vi "HFRR ADV v09 new software.vi"() -> ()   [LabVIEW 2025] (continued)
                        n2272 = local read "EVENT LOG"() -> (w3332:string)
                        n2273 = call "Event Log.vi"("Content"=w3330, "EVENT LOG"=w3332) -> ("EVENT LOG"=w3331:string)  [unwired: 8 in, 1 out]
                        n2274 = local write "EVENT LOG"(w3331) -> ()
                      }
                      frame #22 {
                        n2275 = Wait (ms)(milliseconds to wait=u32 50) -> ()  [unwired: 1 out]
                      }
                      frame #23 {
                        n2276 = local read "NORMAL LOAD"() -> (w3335:dbl)
                        n2277 = Number To Fractional String(number=w3335, precision (6)=i16 2) -> (F-format string=w3336:string)  [unwired: 2 in]
                        n2278 = Concatenate Strings("Applied Load [grams] :" ("Content"), w3336) -> (w3338:string)
                        n2279 = local read "EVENT LOG"() -> (w3340:string)
                        n2280 = call "Event Log.vi"("Content"=w3338, "EVENT LOG"=w3340) -> ("EVENT LOG"=w3339:string)  [unwired: 8 in, 1 out]
                        n2281 = local write "EVENT LOG"(w3339) -> ()
                      }
                      frame #24 {
                        n2282 = Wait (ms)(milliseconds to wait=u32 50) -> ()  [unwired: 1 out]
                      }
                      frame #25 {
                        n2283 = local read "Set Strk"() -> (w3343:dbl)
                        n2284 = Number To Fractional String(number=w3343, precision (6)=i16 2) -> (F-format string=w3344:string)  [unwired: 2 in]
                        n2285 = Concatenate Strings("Set Stroke [mm] :" ("Content"), w3344) -> (w3346:string)
                        n2286 = local read "EVENT LOG"() -> (w3348:string)
                        n2287 = call "Event Log.vi"("Content"=w3346, "EVENT LOG"=w3348) -> ("EVENT LOG"=w3347:string)  [unwired: 8 in, 1 out]
                        n2288 = local write "EVENT LOG"(w3347) -> ()
                      }
                      frame #26 {
                        n2289 = Wait (ms)(milliseconds to wait=u32 50) -> ()  [unwired: 1 out]
                      }
                      frame #27 {
                        n2290 = local read "Set Temp"() -> (w3351:dbl)
                        n2291 = Number To Fractional String(number=w3351, precision (6)=i16 2) -> (F-format string=w3352:string)  [unwired: 2 in]
                        n2292 = Concatenate Strings("Set Temperature [deg C] :" ("Content"), w3352) -> (w3354:string)
                        n2293 = local read "EVENT LOG"() -> (w3356:string)
                        n2294 = call "Event Log.vi"("Content"=w3354, "EVENT LOG"=w3356) -> ("EVENT LOG"=w3355:string)  [unwired: 8 in, 1 out]
                        n2295 = local write "EVENT LOG"(w3355) -> ()
                      }
                      frame #28 {
                        n2296 = Wait (ms)(milliseconds to wait=u32 50) -> ()  [unwired: 1 out]
                      }
                      frame #29 {
                        n2297 = local read "Set Rh"() -> (w3359:dbl)
                        n2298 = Number To Fractional String(number=w3359, precision (6)=i16 2) -> (F-format string=w3360:string)  [unwired: 2 in]
                        n2299 = Concatenate Strings("Set Humidity [%RH] :" ("Content"), w3360) -> (w3362:string)
                        n2300 = local read "EVENT LOG"() -> (w3364:string)
                        n2301 = call "Event Log.vi"("Content"=w3362, "EVENT LOG"=w3364) -> ("EVENT LOG"=w3363:string)  [unwired: 8 in, 1 out]
                        n2302 = local write "EVENT LOG"(w3363) -> ()
                      }
                      frame #30 {
                        n2303 = Wait (ms)(milliseconds to wait=u32 50) -> ()  [unwired: 1 out]
                      }
                      frame #31 {
                        n2304 = local read "test time"() -> (w3367:dbl)
                        n2305 = Number To Fractional String(number=w3367, precision (6)=i16 1) -> (F-format string=w3368:string)  [unwired: 2 in]
                        n2306 = Concatenate Strings("Test Duration [mins] :" ("Content"), w3368) -> (w3370:string)
                        n2307 = local read "EVENT LOG"() -> (w3372:string)
                        n2308 = call "Event Log.vi"("Content"=w3370, "EVENT LOG"=w3372) -> ("EVENT LOG"=w3371:string)  [unwired: 8 in, 1 out]
                        n2309 = local write "EVENT LOG"(w3371) -> ()
                      }
                      frame #32 {
                        w3373 = dbl[] [] ("History Data")
                        w3374 = cluster{"y":dbl, dbl, "y":dbl}[] [] ("History Data")
                        w3375 = FALSE ("Visible")
                        n2310 = property on="Stroke ( mm )" class="WFChart (strict)"("History Data"=w3374) -> ()  [unwired: 2 in, 2 out]
                        n2311 = property on="Humidity ( %RH )" class="WFChart (strict)"("History Data"=w3373) -> ()  [unwired: 2 in, 2 out]
                        n2312 = property on="Temperature ( Deg C )" class="WFChart (strict)"("History Data"=w3373) -> ()  [unwired: 2 in, 2 out]
                        n2313 = property on="Electrical Contact Resistance ( % )" class="WFChart (strict)"("History Data"=w3373) -> ()  [unwired: 2 in, 2 out]
                        n2314 = property on="Coefficient of Friction" class="WFChart (strict)"("History Data"=w3373) -> ()  [unwired: 2 in, 2 out]
                        n2315 = property on="Frictional Force ( N )" class="WFChart (strict)"("History Data"=w3373) -> ()  [unwired: 2 in, 2 out]
                        n2316 = property on="Coefficient of Friction" class="WFChart (strict)"("History Data"=w3373) -> ()  [unwired: 2 in, 2 out]
                        n2317 = property on="Frictional Force ( N )" class="WFChart (strict)"("History Data"=w3373) -> ()  [unwired: 2 in, 2 out]
                        n2318 = property on="Electrical Contact Resistance ( % )" class="WFChart (strict)"("History Data"=w3373) -> ()  [unwired: 2 in, 2 out]
                        n2319 = property on="Humidity ( %RH )" class="WFChart (strict)"("History Data"=w3373) -> ()  [unwired: 2 in, 2 out]
                        n2320 = property on="Stroke ( mm )" class="WFChart (strict)"("History Data"=w3374) -> ()  [unwired: 2 in, 2 out]
                        n2321 = property on="Temperature ( Deg C )" class="WFChart (strict)"("History Data"=w3373) -> ()  [unwired: 2 in, 2 out]
                        n2322 = property on="Service Password Log" class="Str"("Visible"=w3375) -> ()  [unwired: 2 in, 2 out]
                        n2323 = property on="Password 3" class="Clust (strict)"("Visible"=w3375) -> ()  [unwired: 2 in, 2 out]
                      }
                    }
                    "TEST FILE NAM,E SAVED" <- TRUE ("TEST FILE NAM,E SAVED")
                  }
                }
              }
            }
          }
        }
        n2324 = case shown="True" w2679 {
          frame False {
            n2325 = local write "tfalg"(0.0 ("tfalg")) -> ()
          }
          frame True {
            n2326 = local read "tfalg"() -> (w2824:dbl)
            n2327 = Equal?(x=w2824, y=0.0) -> (x = y?=w2825:bool)
            n2328 = case shown="True" w2825 {
              frame False {
              }
              frame True {
                n2329 = local read "Total No. of Tests"() -> (w2828:dbl)
                n2330 = local write "tfalg"(1.0 ("tfalg")) -> ()
                n2331 = local write "acq 2"(FALSE ("acq 2")) -> ()
                n2332 = Wait (ms)(milliseconds to wait=u32 200) -> ()  [unwired: 1 out]
                n2333 = Increment(x=w2828) -> (x+1=w2827:dbl)
                n2334 = local write "Total No. of Tests"(w2827) -> ()
              }
            }
          }
        }
        n2335 = local write "Test \nStatus"(w2685) -> ()
        n2336 = local write "Save"(w2685) -> ()
        n2337 = local read "Main Tab"() -> (w2642:T2)
        n2338 = case shown="True" w2666 {
          tunnel: [FALSE ("RUN") TRUE ("RUN")] -> w2665
          tunnel: [_ 1] -> w2658
          frame False {
          }
          frame True {
          }
        }
        n2339 = In Range and Coerce(upper limit=w2673, x=w2646, lower limit=w2672) -> (In Range?=w2664:bool)  [unwired: 1 out]
        n2340 = In Range and Coerce(upper limit=w2670, x=w2645, lower limit=w2671) -> (In Range?=w2662:bool)  [unwired: 1 out]
        n2341 = case shown="True" w2678 {
          frame False {
            n2342 = local read "Rt 3"() -> (w2806:bool)
            n2343 = case shown="True" w2806 {
              frame False {
              }
              frame True {
                n2344 = local write "Rt 3"(FALSE ("Rt 3")) -> ()
                n2345 = local write "Json End Flg"(TRUE ("Upld AR 2")) -> ()
              }
            }
            "Rt" <- TRUE ("Rt")
            "Rt 2" <- FALSE ("Rt")
          }
          frame True {
            n2346 = local read "Rt"() -> (w2813:bool)
            n2347 = local write "Rt 2"(TRUE ("Rt 2")) -> ()
            n2348 = case shown="True" w2813 {
              frame False {
              }
              frame True {
                w2814 = TRUE ("Upld AR 2")
                n2349 = local write "Rt"(FALSE ("Rt")) -> ()
                n2350 = local write "Upld AR"(w2814) -> ()
                n2351 = local write "Json St Flg"(w2814) -> ()
              }
            }
            "Rt 3" <- TRUE ("Rt 3")
          }
        }
        n2352 = case shown="True" w2664 {
          tunnel: [FALSE ("RUN") TRUE ("RUN")] -> w2663
          tunnel: [_ 2] -> w2657
          frame False {
          }
          frame True {
          }
        }
        n2353 = case shown="True" w2662 {
          tunnel: [FALSE ("RUN") TRUE ("RUN")] -> w2661
          tunnel: [_ 3] -> w2656
          frame False {
          }
          frame True {
          }
        }
        n2354 = case shown="\"Acquire\"" w2642 {
          tunnel: w2644 -> [_ w2875]
          frame Default {
            w2874 = 0.0 ("output")
            n2355 = local write "PID-out"(w2874) -> ()
            n2356 = local write "Frequency ( Hz )"(w2874) -> ()
          }
          frame "Acquire" {
            n2357 = stacked-sequence {
              frame #0 {
                n2358 = local read "Auto Start Test"() -> (w2877:bool)
                n2359 = case shown="True" w2877 {
                  tunnel: "RUN" -> [w2898 w2901]
                  tunnel: [w2898 w2900] -> w2878
                  frame False {
                  }
                  frame True {
                    n2360 = local read "Auto Start Temp"() -> (w2899:bool)
                    n2361 = Or(x=w2901, y=w2899) -> (x .or. y?=w2900:bool)
                  }
                }
                n2362 = local read "clk"() -> (w2897:dbl)
                n2363 = local read "Save"() -> (w2893:bool)
                n2364 = Equal?(x=w2897, y=0.0) -> (x = y?=w2894:bool)
                n2365 = And(x=w2894, y=w2893) -> (x .and. y?=w2895:bool)
                n2366 = Not(x="Engage") -> (.not. x?=w2884:bool)
                n2367 = case shown="True" w2878 {
                  tunnel: [0.0 w2919] -> w2880
                  frame False {
                    (unwired) TRUE ("Visible")
                    n2368 = local read "Auto Start Test"() -> (w2905:bool)
                    n2369 = local write "Start Time"(TRUE ("Start Time")) -> ()
                    n2370 = property on="Stroke 2" class="DigNum (strict)"("Visible"=FALSE) -> ()  [unwired: 2 in, 2 out]
                    n2371 = case shown="False" w2905 {
                      frame False {
                        n2372 = property on="Heater Button" class="Bool (strict)"("DisabledEnum"=T17."Enabled" ("Disabled")) -> ()  [unwired: 2 in, 2 out]
                        n2373 = property on="Humidity" class="Bool (strict)"("DisabledEnum"=T17."Enabled" ("Disabled")) -> ()  [unwired: 2 in, 2 out]
                      }
                      frame True {
                      }
                    }
                    n2374 = case shown="False" "TestCompFlg" {
                      frame False {
                        n2375 = local read "StartFlg"() -> (w2913:bool)
                        n2376 = case shown="True" w2913 {
                          frame False {
                          }
                          frame True {
                            n2377 = flat-sequence {
                              frame #0 {
                                n2378 = local read "EVENT LOG"() -> (w2915:string)
                                n2379 = call "Event Log.vi"("Content"="Test was interrupted", "EVENT LOG"=w2915) -> ("EVENT LOG"=w2916:string)  [unwired: 8 in, 1 out]
                                n2380 = local write "EVENT LOG"(w2916) -> ()
                              }
                              frame #1 {
                                w2918 = FALSE ("StartFlg")
                                n2381 = property on="Heater Button" class="Bool (strict)"("Val(Sgnl)"=FALSE ("Value (Signaling)")) -> ()  [unwired: 2 in, 2 out]
                                n2382 = local write "Heater Button"(w2918) -> ()
                                n2383 = local write "StartFlg"(w2918) -> ()
                                n2384 = local write "Humidity"(w2918) -> ()
                              }
                            }
                          }
                        }
                      }
                      frame True {
                      }
                    }
                    n2385 = local write "String 14"("Test will autostart once parameters reach the set value." ("String 14")) -> ()
                  }
                  frame True {
                    (unwired) FALSE ("Visible")
                    n2386 = property on="Stroke 2" class="DigNum (strict)"("Visible"=TRUE) -> ()  [unwired: 2 in, 2 out]
                    n2387 = property on="STOP 2" class="Bool (strict)"("Disabled"=u8 2) -> ()  [unwired: 2 in, 2 out]
                    n2388 = local write "String 14"(" Running....." ("String 14")) -> ()
                    n2389 = property on="Heater Button" class="Bool (strict)"("DisabledEnum"=T17."Disabled and Grayed Out" ("Disabled")) -> ()  [unwired: 2 in, 2 out]
                    n2390 = property on="Humidity" class="Bool (strict)"("DisabledEnum"=T17."Disabled and Grayed Out" ("Disabled")) -> ()  [unwired: 2 in, 2 out]
                    n2391 = case shown="True" "Start Time" {
                      selector: "Start Time" -> [_ w2938]
                      frame False {
                      }
                      frame True {
                        n2392 = Not(x=w2938) -> (.not. x?=w2937:bool)
                        n2393 = local write "Start Time"(w2937) -> ()
                        n2394 = local read "EVENT LOG"() -> (w2939:string)
                        n2395 = call "Event Log.vi"("Content"="Test in progress", "EVENT LOG"=w2939) -> ("EVENT LOG"=w2941:string)  [unwired: 8 in, 1 out]
                        n2396 = local write "EVENT LOG"(w2941) -> ()
                      }
                    }
                    n2397 = disable-structure shown="Enabled" {
                      disable-tunnel: [w2930 w2936] -> w2919
                      frame Disabled {
                        n2398 = local read "Set Hz"() -> (w2933:dbl)
                        n2399 = call <vilib>:"Uniform White Noise Waveform.vi"() -> ("signal out"=w2932:waveform(dbl))  [unwired: 10 in, 1 out]
                        n2400 = Random Number (0-1)() -> (number: 0 to 1=w2929:dbl)
                        n2401 = Add(x=w2933, y=w2932) -> (x+y=w2931:waveform(dbl))
                        n2402 = Multiply(x=ext 0.01 ("y"), y=w2929) -> (x*y=w2927:ext)
                        n2403 = Multiply(x=w2931, y=w2927) -> (x*y=w2930:waveform(ext))
                      }
                      frame Enabled {
                        n2404 = call-poly <vilib>:"Random Number (Range).vi"("lower bound (0)"=49.89, "upper bound (100)"=50.8) -> ("number"=w2936:dbl)  [unwired: 9 in]
                      }
                    }
                    "StartFlg" <- TRUE ("StartFlg")
                  }
                }
                n2405 = case shown="True" w2895 {
                  frame False {
                  }
                  frame True {
                    n2406 = local write "clk"(10.0 ("clk")) -> ()
                    n2407 = Get Date/Time In Seconds() -> (seconds since 1Jan1904=w2944:timestamp)
                    n2408 = To Double Precision Float(number=w2944) -> (double precision float=w2942:dbl)
                    n2409 = local write "acq timer"(w2942) -> ()
                    n2410 = local write "act save time"(w2942) -> ()
                  }
                }
                n2411 = call "Elapsed Time"("Time Target (s)"="Countdown", "Reset"=w2884) -> ("Elapsed Time (s)"=w2889:dbl, "Time has Elapsed"=w2887:bool)  [unwired: 10 in, 6 out]
                "Countdown 2" <- w2889
                n2412 = Subtract(x=w2889, y=2.0) -> (x-y=w2892:dbl)
                n2413 = Less?(x=w2892, y="Countdown") -> (x < y?=w2890:bool)
                n2414 = And(x=w2890, y=w2887) -> (x .and. y?=w2886:bool)
                n2415 = case shown="True" w2886 {
                  frame False {
                  }
                  frame True {
                    (unwired) dbl[] [] ("History Data")
                    n2416 = local write "Engage"(FALSE ("Engage")) -> ()
                    n2417 = local write "RUN"(TRUE ("RUN")) -> ()
                    n2418 = local read "Humidity ( %RH )"() -> (→"Rh Before":dbl)
                  }
                }
                n2419 = local read "Test \nStatus"() -> (w2882:bool)
                n2420 = Select(t=w2880, s=w2882, f=0.0) -> (s? t:f=w2881:dbl)
                n2421 = local write "Frequency ( Hz )"(w2881) -> ()
              }
              frame #1 {
                w2967 = 1000000.0 ("x")
                # "HC;1/0\nST;VALUE"
                # "Elapsed time\ncof\nstroke\nAir temp\nTemp\nHumidity"
                # "acq timer\n\nact save time"
                # "convert to microseconds"
                n2422 = local read "COUNT"() -> (w2950:i32)
                n2423 = local read "Rate"() -> (w2963:dbl)
                n2424 = Divide(x=w2967, y=w2963) -> (x/y=w2968:dbl)
                n2425 = Greater Or Equal?(x=w2950, y=250) -> (x >= y?=w2949:bool)
                n2426 = Get Date/Time In Seconds() -> (seconds since 1Jan1904=w2970:timestamp)
                n2427 = case shown="True" w2949 {
                  frame False {
                    n2428 = local read "COUNT"() -> (w2971:i32)
                    n2429 = Increment(x=w2971) -> (x+1=w2972:i32)
                    n2430 = local write "COUNT"(w2972) -> ()
                  }
                  frame True {
                    n2431 = local write "COUNT"(0 ("COUNT")) -> ()
                  }
                }
                n2432 = local read "Samplingtime 2"() -> (w2948:dbl)
                n2433 = local read "act save time"() -> (w2965:dbl)
                n2434 = Divide(x=w2968, y=w2967) -> (x/y=w2966:dbl)
                n2435 = To Double Precision Float(number=w2970) -> (double precision float=w2959:dbl)
                n2436 = Add(x=w2965, y=w2948) -> (x+y=w2964:dbl)
                n2437 = local read "acq timer"() -> (w2969:dbl)
                n2438 = local read "COUNT"() -> (w2952:i32)
                n2439 = Greater Or Equal?(x=w2959, y=w2964) -> (x >= y?=w2947:bool)
                n2440 = Multiply(x=w2966, y=w2952) -> (x*y=w2958:dbl)
                n2441 = Subtract(x=w2959, y=w2969) -> (x-y=w2961:dbl)
                n2442 = local read "Save"() -> (w2962:bool)
                n2443 = Add(x=w2961, y=w2958) -> (x+y=w2945:dbl)
                "Elapsed time 3" <- w2945
                n2444 = And(x=w2947, y=w2962) -> (x .and. y?=w2960:bool)
                n2445 = Divide(x=w2945, y=60.0) -> (x/y=w2956:dbl)
                n2446 = local read "Test \nStatus"() -> (w2946:bool)
                n2447 = local read "clk"() -> (w2953:dbl)
                n2448 = Equal?(x=w2953, y=10.0) -> (x = y?=w2955:bool)
                n2449 = case shown="True" w2960 {
                  tunnel: w2959 -> [_ w3081]
                  tunnel: [FALSE ("Boolean 2") TRUE ("Boolean 2")] -> _
                  frame False {
                  }
                  frame True {
                    w3035 = ";" ("Substring")
                    # "Pid out/\nFreq response value"
                    n2450 = local write "act save time"(w3081) -> ()
                    n2451 = local read "FILE"() -> (w3029:string)
                    n2452 = call "file check.vi"("file name in"=w3029) -> ("error out"=w3032:errorcluster, "file name out"=w3027:string)  [unwired: 9 in]
                    n2453 = call "FILE PATH CREATION.vi"("error in"=w3032, "FILE NAME :"=w3027) -> ("FILE OUT"=w3030:path)  [unwired: 8 in, 1 out]
                    n2454 = Concatenate Strings(w3027, ".dgf" ("Substring")) -> (w3031:string)
                    n2455 = local read "FF 2"() -> (→"Frictional Force ( N )" →"Frictional Force ( N )":dbl)
                    n2456 = Build Path(base path=w3030, name or relative path=w3031) -> (appended path=w3026:path)
                    n2457 = local read "COF 2"() -> (w3040:dbl)
                    "cof" <- w3040
                    "Coefficient of Friction" <- w3040
                    "COF 4" <- w3040
                    "Coefficient of Friction" <- w3040
                    n2458 = local read "LVDT STROKE"() -> (w3024:dbl)
                    n2459 = local read "Add up Stroke"() -> (w3022:dbl)
                    n2460 = local read "TEMP"() -> (w3043:dbl)
                    "Temp" <- w3043
                    "Temperature ( Deg C )" <- w3043
                    n2461 = local read "Humidity ( %RH )"() -> (w3042:dbl)
                    "Humidity ( %RH )" <- w3042
                    "Humidity ( %RH )" <- w3042
                    n2462 = local read "Frequency ( Hz )"() -> (w3049:dbl)
                    n2463 = local read "Elapsed time"() -> (w3074:dbl)
                    n2464 = local read "AIR TEMP"() -> (w3047:dbl)
                    n2465 = local read "PID-out"() -> (w3052:dbl)
                    n2466 = Subtract(x=w3024, y=w3022) -> (x-y=w3023:dbl)
                    n2467 = Absolute Value(x=w3023) -> (abs(x)=w3021:dbl)
                    n2468 = local write "Temperature ( Deg C )"(w3043) -> ()
                    n2469 = Number To Fractional String(number=w3021, width (-)=i16 9 ("precision (6)"), precision (6)=i16 6) -> (F-format string=w3067:string)  [unwired: 1 in]
                    n2470 = Number To Fractional String(number=w3047, width (-)=i16 9 ("precision (6)"), precision (6)=i16 3) -> (F-format string=w3066:string)  [unwired: 1 in]
                    n2471 = Number To Fractional String(number=w3043, width (-)=i16 9 ("precision (6)"), precision (6)=i16 3) -> (F-format string=w3063:string)  [unwired: 1 in]
                    n2472 = Number To Fractional String(number=w3042, width (-)=i16 9 ("precision (6)"), precision (6)=i16 3) -> (F-format string=w3060:string)  [unwired: 1 in]
                    n2473 = Number To Fractional String(number=0.0, width (-)=i16 9 ("precision (6)"), precision (6)=i16 3) -> (F-format string=w3057:string)  [unwired: 1 in]
                    n2474 = Number To Fractional String(number=w3052, width (-)=i16 9 ("precision (6)"), precision (6)=i16 3) -> (F-format string=w3053:string)  [unwired: 1 in]
                    n2475 = Number To Fractional String(number=w3049, width (-)=i16 9 ("precision (6)"), precision (6)=i16 3) -> (F-format string=w3048:string)  [unwired: 1 in]
                    n2476 = Number To Fractional String(number=w3040, width (-)=i16 9 ("precision (6)"), precision (6)=i16 6) -> (F-format string=w3075:string)  [unwired: 1 in]
                    n2477 = Number To Fractional String(number=w3074, width (-)=i16 14 ("precision (6)"), precision (6)=i16 3) -> (F-format string=w3076:string)  [unwired: 1 in]
                    n2478 = Bundle("y"=1.02, w3021, "y"=0.98) -> (w3041:cluster{"y":dbl, dbl, "y":dbl})  [unwired: 1 in]
                    n2479 = Number To Fractional String(number="Ambient Humidity :", width (-)=i16 9 ("precision (6)"), precision (6)=i16 6) -> (F-format string=w3033:string)  [unwired: 1 in]
                    n2480 = local read "RUN"() -> (w3039:bool)
                    n2481 = case shown="True" w3039 {
                      tunnel: w3041 -> [_ w3086]
                      tunnel: w3021 -> [_ w3085]
                      tunnel: w3021 -> [_ w3083]
                      tunnel: w3021 -> [_ w3084]
                      frame False {
                      }
                      frame True {
                        "Stroke ( mm )" <- w3086
                        "Stroke ( mm )" <- w3086
                        "Stroke 4" <- w3085
                        "Stroke 3" <- w3083
                        "Stroke 2" <- w3084
                        "measured_stroke" <- w3083
                      }
                    }
                    n2482 = Concatenate Strings(w3076, w3035, w3075, w3035, w3067, w3035, w3066, w3035, w3063, w3035, w3060, w3035, w3057, w3035, w3053, w3035, w3048, w3035, w3033, "\r") -> (w3073:string)
                    n2483 = call <vilib>:"Write Characters To File.vi"("append to file? (new file:F)"=TRUE, "character string"=w3073, "file path (dialog if empty)"=w3026) -> ()  [unwired: 2 in, 1 out]
                    "refresh flag" <- TRUE ("refresh flag")
                  }
                }
                n2484 = case shown="True" w2946 {
                  tunnel: w2956 -> [_ w2982]
                  tunnel: w2961 -> [_ w2992]
                  tunnel: [0.0 w2988] -> _
                  tunnel: w2955 -> [_ w2987]
                  tunnel: [0.0 w2986] -> _
                  tunnel: w2945 -> [_ w2986]
                  tunnel: w2959 -> [w2975 _]
                  frame False {
                    n2485 = local write "acq timer"(w2975) -> ()
                    n2486 = local write "Test Duration Status"(0.0 ("Test Duration Status")) -> ()
                  }
                  frame True {
                    n2487 = local read "Set Hz"() -> (w2989:dbl)
                    n2488 = local write "Elapsed time"(w2982) -> ()
                    n2489 = local read "test time"() -> (w2981:dbl)
                    n2490 = Multiply(x=w2992, y=w2989) -> (x*y=w2991:dbl)
                    n2491 = case shown="False" w2987 {
                      tunnel: w2991 -> [w2993 _]
                      tunnel: [w2993 1.0] -> w2988
                      frame False {
                        n2492 = local write "Cycles elapsed"(w2993) -> ()
                      }
                      frame True {
                      }
                    }
                    n2493 = Greater?(x=w2982, y=w2981) -> (0:w2990:bool)
                    n2494 = Subtract(x=w2981, y=w2982) -> (x-y=w2980:dbl)
                    "time" <- w2980
                    n2495 = Multiply(x=w2980, y=60.0) -> (x*y=w2979:dbl)
                    n2496 = local write "Time Remaining"(w2979) -> ()
                    n2497 = local write "Remaining Time"(w2979) -> ()
                    n2498 = case shown="True" w2990 {
                      frame False {
                      }
                      frame True {
                        n2499 = stacked-sequence {
                          frame #0 {
                            w2998 = T17."Enabled" ("Disabled")
                            w2997 = FALSE ("TEST FILE NAM,E SAVED")
                            w2999 = "" ("FILE")
                            w3000 = TRUE ("Visible")
                            n2500 = local write "Humidity"(FALSE ("Humidity")) -> ()
                            n2501 = local write "RUN"(FALSE ("OK Button 2")) -> ()
                            n2502 = local write "Heater Button"(FALSE ("Heater Button")) -> ()
                            n2503 = local write "Auto Start Test"(FALSE ("Auto Start Test")) -> ()
                            n2504 = local write "TestCompFlg"(TRUE ("StpFlg")) -> ()
                            n2505 = local read "Humidity ( %RH )"() -> (→"Rh After":dbl)
                            n2506 = property on="STOP 2" class="Bool (strict)"("Disabled"=u8 0) -> ()  [unwired: 2 in, 2 out]
                            n2507 = local read "EVENT LOG"() -> (w3005:string)
                            n2508 = call "Event Log.vi"("Content"="Test Completed", "EVENT LOG"=w3005) -> ("EVENT LOG"=w3004:string)  [unwired: 8 in, 1 out]
                            n2509 = property on="RUN" class="Bool (strict)"("Visible"=w3000) -> ()  [unwired: 2 in, 2 out]
                            n2510 = property on="Auto Start Test" class="Bool (strict)"("Visible"=w3000) -> ()  [unwired: 2 in, 2 out]
                            n2511 = local write "Batch Ref Num :"(w2999) -> ()
                            n2512 = local write "FILE"(w2999) -> ()
                            n2513 = local write "EVENT LOG"(w3004) -> ()
                            n2514 = local write "TEST FILE NAM,E SAVED"(w2997) -> ()
                            n2515 = local write "Fuel Discription :"(w2999) -> ()
                            n2516 = local write "START TEMP"(w2997) -> ()
                            n2517 = local write "Remarks :"(w2999) -> ()
                            n2518 = local write "Main Dashboard Buttons"(T1."Imaging" ("Main Dashboard Buttons")) -> ()
                            n2519 = local write "Main Tab"(T2."Adv Scar" ("Main Tab")) -> ()
                            n2520 = property on="FRICVALZ 2" class="Bool (strict)"("DisabledEnum"=w2998) -> ()  [unwired: 2 in, 2 out]
                            n2521 = property on="FRICVALZ 3" class="Bool (strict)"("DisabledEnum"=w2998) -> ()  [unwired: 2 in, 2 out]
                            n2522 = property on="FRICVALZ 4" class="Bool (strict)"("DisabledEnum"=w2998) -> ()  [unwired: 2 in, 2 out]
                          }
                          frame #1 {
                            n2523 = Wait (ms)(milliseconds to wait=u32 1500) -> ()  [unwired: 1 out]
                          }
                          frame #2 {
                            n2524 = local write "Command"("VC;0") -> ()
                          }
                          frame #3 {
                            n2525 = Wait (ms)(milliseconds to wait=u32 1500) -> ()  [unwired: 1 out]
                          }
                          frame #4 {
                            n2526 = local write "Command"("VC;0") -> ()
                          }
                          frame #5 {
                            n2527 = Wait (ms)(milliseconds to wait=u32 1500) -> ()  [unwired: 1 out]
                          }
                          frame #6 {
                            n2528 = local write "Command"("ST;0") -> ()
                          }
                          frame #7 {
                            n2529 = local write "measured_stroke"(0.0 ("measured_stroke")) -> ()
                            n2530 = Wait (ms)(milliseconds to wait=u32 1500) -> ()  [unwired: 1 out]
                          }
                          frame #8 {
                            n2531 = local write "Command"("HE;0") -> ()
                          }
                        }
                      }
                    }
                    n2532 = Divide(x=w2982, y=w2981) -> (x/y=w2985:dbl)
                    n2533 = Multiply(x=w2985, y=100.0) -> (x*y=w2983:dbl)
                    n2534 = local write "Test Duration Status"(w2983) -> ()
                  }
                }
              }
              frame #2 {
                n2535 = case shown="True" "Heater Button" {
                  tunnel: [0.0 ("output") w3109] -> w3087
                  frame False {
                    w3090 = TRUE ("tmpchk")
                    n2536 = local read "TEMP"() -> (w3091:dbl)
                    n2537 = local write "Temp ini"(w3091) -> ()
                    n2538 = local write "Reset 4"(w3090) -> ()
                    n2539 = local write "tmpchk"(w3090) -> ()
                    n2540 = local write "reinit"(TRUE ("reinit")) -> ()
                    n2541 = local write "manual temp log"(TRUE ("manual temp log")) -> ()
                  }
                  frame True {
                    # "Logic to turn off\nthe heater when \ntemp is not rising.\nTime - 60 sec\nDelta t- 5°c"
                    n2542 = local read "Temp ini"() -> (w3098:dbl)
                    n2543 = local read "Auto Start Test"() -> (w3094:bool)
                    n2544 = Less?(x=w3098, y=53.0) -> (x < y?=w3096:bool)
                    n2545 = case shown="False" w3094 {
                      frame False {
                        n2546 = local read "Set Temp"() -> (w3118:dbl)
                        n2547 = local read "TEMP"() -> (w3117:dbl)
                        n2548 = Subtract(x=w3118, y=w3117) -> (x-y=w3116:dbl)
                        n2549 = Absolute Value(x=w3116) -> (abs(x)=w3115:dbl)
                        n2550 = Less?(x=w3115, y=0.5) -> (x < y?=w3113:bool)
                        n2551 = case shown="True" w3113 {
                          tunnel: "manual temp log" -> [_ w3119]
                          frame False {
                          }
                          frame True {
                            n2552 = case shown="True" w3119 {
                              selector: w3119 -> [_ w3120]
                              frame False {
                              }
                              frame True {
                                # "#Event log"
                                n2553 = Not(x=w3120) -> (.not. x?=w3121:bool)
                                n2554 = local write "manual temp log"(w3121) -> ()
                                n2555 = local read "EVENT LOG"() -> (w3124:string)
                                n2556 = call "Event Log.vi"("Content"="Target Temperature reached", "EVENT LOG"=w3124) -> ("EVENT LOG"=w3123:string)  [unwired: 8 in, 1 out]
                                n2557 = local write "EVENT LOG"(w3123) -> ()
                              }
                            }
                          }
                        }
                      }
                      frame True {
                        n2558 = local write "manual temp log"(TRUE ("manual temp log")) -> ()
                      }
                    }
                    n2559 = And(x="tmpchk", y=w3096) -> (x .and. y?=w3099:bool)
                    n2560 = case shown="True" w3099 {
                      frame False {
                      }
                      frame True {
                        n2561 = call "Elapsed Time8"("Time Target (s)"=300.0, "Reset"="Reset 4") -> ("Time has Elapsed"=w3126:bool)  [unwired: 10 in, 7 out]
                        n2562 = flat-sequence {
                          tunnel: w3126 -> [_]
                          frame #0 {
                            n2563 = local write "Reset 4"(FALSE ("Reset 4")) -> ()
                          }
                        }
                        n2564 = case shown="True" w3126 {
                          frame False {
                          }
                          frame True {
                            n2565 = local read "Temp ini"() -> (w3133:dbl)
                            n2566 = Add(x=w3133, y=5.0) -> (x+y=w3131:dbl)
                            n2567 = local read "TEMP"() -> (w3134:dbl)
                            n2568 = Greater?(x=w3134, y=w3131) -> (0:w3132:bool)
                            n2569 = case shown="False" w3132 {
                              frame False {
                                n2570 = local write "Heater Button"(FALSE ("Heater Button")) -> ()
                              }
                              frame True {
                                n2571 = local write "tmpchk"(FALSE ("tmpchk")) -> ()
                              }
                            }
                          }
                        }
                      }
                    }
                    n2572 = local read "Set Temp"() -> (w3107:dbl)
                    n2573 = local read "TEMP"() -> (w3101:dbl)
                    n2574 = call-poly <vilib>:"PID.vi"("reinitialize? (F)"="reinit", "dt (s)"=-1.0, "process variable"=w3101, "setpoint"=w3107) -> ("output"=w3104:dbl)  [unwired: 6 in, 1 out]
                    n2575 = Subtract(x=w3107, y=w3101) -> (x-y=w3108:dbl)
                    n2576 = Add(x=w3107, y=0.5) -> (x+y=w3105:dbl)
                    n2577 = Greater Or Equal?(x=w3101, y=w3105) -> ()  [unwired: 1 out]
                    n2578 = Select(t=0.0, s=FALSE, f=w3104) -> (s? t:f=w3103:dbl)
                    "PID output" <- w3103
                    n2579 = flat-sequence {
                      tunnel: w3103 -> [w3137]
                      tunnel: [w3137] -> w3109
                      frame #0 {
                        n2580 = local write "reinit"(FALSE ("reinit")) -> ()
                      }
                    }
                    n2581 = Bundle(w3108, "output"=w3103, "TEMP"=w3101) -> ()  [unwired: 1 in, 1 out]
                  }
                }
                "PID-out" <- w3087
              }
              frame #3 {
                n2582 = local read "TEMP"() -> (w3139:dbl)
                n2583 = Greater Or Equal?(x=w3139, y="Set Temp 2") -> (x >= y?=w3144:bool)
                n2584 = case shown="True" w3144 {
                  tunnel: [FALSE TRUE] -> w3142
                  frame False {
                  }
                  frame True {
                  }
                }
                "Status 13" <- w3142
                n2585 = And(x=w3142, y="trip1 8") -> (x .and. y?=w3141:bool)
                n2586 = case shown="True" w3141 {
                  frame False {
                    n2587 = local write "Heater Trip Temp"(TRUE ("Heater Trip Temp")) -> ()
                  }
                  frame True {
                    w3147 = FALSE ("OK Button 2")
                    n2588 = case shown="True" "Heater Trip Temp" {
                      selector: "Heater Trip Temp" -> [_ w3149]
                      frame False {
                      }
                      frame True {
                        n2589 = Not(x=w3149) -> (.not. x?=w3148:bool)
                        n2590 = local read "EVENT LOG"() -> (w3152:string)
                        n2591 = local write "Heater Trip Temp"(w3148) -> ()
                        n2592 = call "Event Log.vi"("Content"="Heater Trip", "EVENT LOG"=w3152) -> ("EVENT LOG"=w3151:string)  [unwired: 8 in, 1 out]
                        n2593 = local write "EVENT LOG"(w3151) -> ()
                      }
                    }
                    n2594 = local write "RUN"(w3147) -> ()
                    n2595 = property on="Auto Start Test" class="Bool (strict)"("Value"=w3147) -> ()  [unwired: 2 in, 2 out]
                    n2596 = local write "Heater Button"(w3147) -> ()
                  }
                }
              }
            }
            n2597 = case shown="False" w2875 {
              frame False {
                n2598 = disable-structure shown="Disabled" {
                  frame Disabled {
                    n2599 = stacked-sequence {
                      frame #0 {
                        n2600 = local write "RUN"(FALSE ("OK Button 2")) -> ()
                      }
                      frame #1 {
                      }
                    }
                  }
                  frame Enabled {
                  }
                }
              }
              frame True {
              }
            }
          }
        }
        n2601 = local read "airtempflg"() -> (w2667:bool)
        n2602 = Or(x=w2667, y=w2665) -> (x .or. y?=w2668:bool)
        n2603 = Insert Into Array(array=string[] ["Air Temperature has reached set value,", "Humidity has reached set value,", "Sample Temperaturehas reached set value,", ""], index=0, new element="") -> (w2653:string[])
        n2604 = Build Array(w2658, w2657, w2656) -> (w2654:i32[])
        n2605 = disable-structure shown="Disabled" {
          disable-tunnel: w2668 -> [w2745 _]
          disable-tunnel: w2663 -> [w2744 _]
          disable-tunnel: w2661 -> [w2743 _]
          frame Disabled {
            n2606 = Compound Arithmetic op=AND(w2745, w2744, w2743) -> ()  [unwired: 1 out]
            n2607 = case shown="True" {
              selector: _ -> [_ _]
              frame False {
              }
              frame True {
                w2746 = FALSE ("autostrtflg")
                n2608 = local write "RUN"(TRUE ("RUN")) -> ()
                n2609 = local write "autostrtflg"(w2746) -> ()
                n2610 = local write "autostart"(w2746) -> ()
                n2611 = local write "String 14"(" Running....." ("String 14")) -> ()
              }
            }
          }
          frame Enabled {
          }
        }
        n2612 = for {
          tunnel: w2654 -> [w2796] mode=indexing
          tunnel: w2653 -> [w2795]
          shift-right: [w2792] -> w2652
          shift-left: "" -> [w2794]
          n2613 = Index Array(array=w2795, index=w2796) -> (element=w2793:string)
          n2614 = Concatenate Strings(w2793, w2794) -> (w2792:string)
        }
        n2615 = local write "autostart 2"(w2652) -> ()
        n2616 = local read "Reset Graph"() -> (w2641:bool)
        n2617 = case shown="True" w2641 {
          selector: w2641 -> [_ w2695]
          frame False {
          }
          frame True {
            w2709 = 0.0 ("X Scale.Range:Maximum")
            n2618 = Not(x=w2695) -> (.not. x?=w2694:bool)
            n2619 = local write "Reset Graph"(w2694) -> ()
            n2620 = property on="Electrical Contact Resistance ( % )" class="WFChart (strict)"("XScale.Maximum"=600.0 ("X Scale.Range:Maximum"), "XScale.Minimum"=0.0 ("X Scale.Range:Minimum"), "YScale.Maximum"=100.0 ("Y Scale.Range:Maximum"), "YScale.Minimum"=0.0 ("Y Scale.Range:Minimum")) -> ()  [unwired: 2 in, 2 out]
            n2621 = property on="Frictional Force ( N )" class="WFChart (strict)"("XScale.Maximum"=600.0 ("X Scale.Range:Maximum"), "XScale.Minimum"=0.0 ("X Scale.Range:Minimum"), "YScale.Maximum"=100.0 ("Y Scale.Range:Maximum"), "YScale.Minimum"=0.0 ("Y Scale.Range:Minimum")) -> ()  [unwired: 2 in, 2 out]
            n2622 = property on="Temperature ( Deg C )" class="WFChart (strict)"("XScale.Maximum"=600.0 ("X Scale.Range:Maximum"), "XScale.Minimum"=0.0 ("X Scale.Range:Minimum"), "YScale.Maximum"=100.0 ("Y Scale.Range:Maximum"), "YScale.Minimum"=0.0 ("Y Scale.Range:Minimum")) -> ()  [unwired: 2 in, 2 out]
            n2623 = property on="Humidity ( %RH )" class="WFChart (strict)"("XScale.Maximum"=600.0 ("X Scale.Range:Maximum"), "XScale.Minimum"=0.0 ("X Scale.Range:Minimum"), "YScale.Maximum"=100.0 ("Y Scale.Range:Maximum"), "YScale.Minimum"=0.0 ("Y Scale.Range:Minimum")) -> ()  [unwired: 2 in, 2 out]
            n2624 = property on="Stroke ( mm )" class="WFChart (strict)"("XScale.Maximum"=600.0 ("X Scale.Range:Maximum"), "XScale.Minimum"=0.0 ("X Scale.Range:Minimum"), "YScale.Maximum"=100.0 ("Y Scale.Range:Maximum"), "YScale.Minimum"=0.0 ("Y Scale.Range:Minimum")) -> ()  [unwired: 2 in, 2 out]
            n2625 = property on="Coefficient of Friction" class="WFChart (strict)"("XScale.Maximum"=600.0 ("X Scale.Range:Maximum"), "XScale.Minimum"=0.0 ("X Scale.Range:Minimum"), "YScale.Maximum"=100.0 ("Y Scale.Range:Maximum"), "YScale.Minimum"=0.0 ("Y Scale.Range:Minimum")) -> ()  [unwired: 2 in, 2 out]
            n2626 = property on="Electrical Contact Resistance ( % )" class="WFChart (strict)"("XScale.Minimum"=0.0 ("X Scale.Range:Minimum"), "XScale.Maximum"=600.0 ("X Scale.Range:Maximum"), "YScale.Minimum"=0.0 ("Y Scale.Range:Minimum"), "YScale.Maximum"=100.0 ("Y Scale.Range:Maximum")) -> ()  [unwired: 2 in, 2 out]
            n2627 = property on="Temperature ( Deg C )" class="WFChart (strict)"("XScale.Minimum"=0.0 ("X Scale.Range:Minimum"), "XScale.Maximum"=600.0 ("X Scale.Range:Maximum"), "YScale.Minimum"=0.0 ("Y Scale.Range:Minimum"), "YScale.Maximum"=100.0 ("Y Scale.Range:Maximum")) -> ()  [unwired: 2 in, 2 out]
            n2628 = property on="Coefficient of Friction" class="WFChart (strict)"("XScale.Minimum"=0.0 ("X Scale.Range:Minimum"), "XScale.Maximum"=600.0 ("X Scale.Range:Maximum"), "YScale.Maximum"=1.0 ("X Scale.Range:Minimum"), "YScale.Minimum"=0.0 ("X Scale.Range:Minimum")) -> ()  [unwired: 2 in, 2 out]
            n2629 = property on="Frictional Force ( N )" class="WFChart (strict)"("XScale.Maximum"=600.0 ("X Scale.Range:Maximum"), "XScale.Minimum"=w2709, "YScale.Maximum"=10.0 ("Y Scale.Range:Maximum"), "YScale.Minimum"=w2709) -> ()  [unwired: 2 in, 2 out]
            n2630 = property on="Stroke ( mm )" class="WFChart (strict)"("XScale.Maximum"=600.0 ("X Scale.Range:Maximum"), "XScale.Minimum"=0.0 ("X Scale.Range:Minimum"), "YScale.Maximum"=100.0 ("Y Scale.Range:Maximum"), "YScale.Minimum"=0.0 ("Y Scale.Range:Minimum")) -> ()  [unwired: 2 in, 2 out]
            n2631 = property on="Humidity ( %RH )" class="WFChart (strict)"("XScale.Maximum"=600.0 ("X Scale.Range:Maximum"), "XScale.Minimum"=0.0 ("X Scale.Range:Minimum"), "YScale.Maximum"=100.0 ("Y Scale.Range:Maximum"), "YScale.Minimum"=0.0 ("Y Scale.Range:Minimum")) -> ()  [unwired: 2 in, 2 out]
          }
        }
      }
      frame "Compare Files" {
        # "Elapsed time\ncof\nstroke\nAir temp\nTemp\nHumidity"
        n2632 = case shown="True" "RSTV1 2" {
          frame False {
          }
          frame True {
            n2633 = property on="Humidity ( %RH )" class="XYGraph (strict)"("Y Scale.Display Format:Precision"=u8 0 ("Y Scale.Format & Precision:Precision")) -> ()  [unwired: 2 in, 2 out]
            n2634 = property on="Humidity ( %RH )" class="XYGraph (strict)"("X Scale.Range:Minimum"=0.0, "X Scale.Range:Maximum"=75.0, "Y Scale.Range:Minimum"=48.0, "Y Scale.Range:Maximum"=58.0) -> ()  [unwired: 2 in, 2 out]
          }
        }
        n2635 = case shown="True" "RST CP 2" {
          frame False {
          }
          frame True {
            n2636 = property on="XY Graph 13" class="XYGraph (strict)"("Y Scale.Display Format:Precision"=u8 0 ("Y Scale.Format & Precision:Precision")) -> ()  [unwired: 2 in, 2 out]
            n2637 = property on="XY Graph 13" class="XYGraph (strict)"("X Scale.Range:Minimum"=0.0, "X Scale.Range:Maximum"=75.0, "Y Scale.Range:Minimum"=0.0, "Y Scale.Range:Maximum"=100.0) -> ()  [unwired: 2 in, 2 out]
          }
        }
        n2638 = case shown="True" "RST CP" {
          frame False {
          }
          frame True {
            n2639 = property on="Sample Temperature ( °C )" class="XYGraph (strict)"("Y Scale.Display Format:Precision"=u8 2 ("Y Scale.Format & Precision:Precision")) -> ()  [unwired: 2 in, 2 out]
            n2640 = property on="Sample Temperature ( °C )" class="XYGraph (strict)"("X Scale.Range:Minimum"=0.0, "X Scale.Range:Maximum"=75.0, "Y Scale.Range:Minimum"=58.0, "Y Scale.Range:Maximum"=62.0) -> ()  [unwired: 2 in, 2 out]
          }
        }
        n2641 = case shown="True" "RSTV1 3" {
          frame False {
          }
          frame True {
            n2642 = property on="Air Temperature  ( °C )" class="XYGraph (strict)"("Y Scale.Display Format:Precision"=u8 2 ("Y Scale.Format & Precision:Precision")) -> ()  [unwired: 2 in, 2 out]
            n2643 = property on="Air Temperature  ( °C )" class="XYGraph (strict)"("X Scale.Range:Minimum"=0.0 ("Y Scale.Range:Minimum"), "X Scale.Range:Maximum"=75.0 ("Y Scale.Range:Maximum"), "Y Scale.Range:Minimum"=20.0 ("X Scale.Range:Minimum"), "Y Scale.Range:Maximum"=26.0 ("X Scale.Range:Maximum")) -> ()  [unwired: 2 in, 2 out]
          }
        }
        n2644 = case shown="True" "RSTV1 4" {
          frame False {
          }
          frame True {
            n2645 = property on="Stroke ( mm )" class="XYGraph (strict)"("Y Scale.Display Format:Precision"=u8 2 ("Y Scale.Format & Precision:Precision")) -> ()  [unwired: 2 in, 2 out]
            n2646 = property on="Stroke ( mm )" class="XYGraph (strict)"("X Scale.Range:Minimum"=0.0 ("Y Scale.Range:Maximum"), "X Scale.Range:Maximum"=75.0 ("X Scale.Range:Minimum"), "Y Scale.Range:Minimum"=0.98, "Y Scale.Range:Maximum"=1.02) -> ()  [unwired: 2 in, 2 out]
          }
        }
        n2647 = case shown="True" "rstv2" {
          frame False {
          }
          frame True {
            n2648 = property on="Coefficient Of Friction" class="XYGraph (strict)"("Y Scale.Display Format:Precision"=u8 3 ("Y Scale.Format & Precision:Precision")) -> ()  [unwired: 2 in, 2 out]
            n2649 = property on="Coefficient Of Friction" class="XYGraph (strict)"("X Scale.Range:Minimum"=0.0 ("Y Scale.Range:Maximum"), "X Scale.Range:Maximum"=75.0, "Y Scale.Range:Minimum"=0.0, "Y Scale.Range:Maximum"=1.0 ("X Scale.Range:Minimum")) -> ()  [unwired: 2 in, 2 out]
          }
        }
        n2650 = case shown="True" "RST CP 3" {
          frame False {
          }
          frame True {
            n2651 = property on="Air Temp ( °C ) vs Humidity ( % RH )" class="XYGraph (strict)"("X Scale.Range:Minimum"=18.0, "X Scale.Range:Maximum"=28.0 ("X Scale.Range:Minimum"), "Y Scale.Range:Minimum"=30.0 ("X Scale.Range:Minimum"), "Y Scale.Range:Maximum"=70.0 ("X Scale.Range:Minimum")) -> ()  [unwired: 2 in, 2 out]
          }
        }
        n2652 = case shown="True" "OPEN 1" {
          frame False {
          }
          frame True {
            (unwired) 0  # existing file
            w3428 = "Choose a datalog file to open"  # prompt
            n2653 = local write "OPEN 1"(FALSE ("OPEN 1")) -> ()
            n2654 = String To Path(string="C:\\LAB-IQ\\Data\\") -> (path=w3413:path)
            n2655 = File Dialog(6:"*.dgf" ("pattern"), 7:w3428, 11:w3413) -> (0:w3411:errorcluster, 3:w3419:path)  [unwired: 4 in, 2 out]
            n2656 = Unbundle(w3411) -> ()  [unwired: 3 out]
            n2657 = Strip Path(path=w3419) -> (name=w3418:string)  [unwired: 1 out]
            n2658 = Path To String(path=w3419) -> (string=w3414:string)
            "string1" <- w3414
            n2659 = Match Pattern(string=w3418, regular expression=".dgf") -> (before substring=→"String Control":string)  [unwired: 1 in, 3 out]
            n2660 = Match Pattern(string=w3414, regular expression=".dgf" ("substring (\"\")")) -> (before substring=w3424:string)  [unwired: 1 in, 3 out]
            n2661 = Concatenate Strings(w3424, ".duf" ("Substring")) -> (w3420:string)
            n2662 = String To Path(string=w3420) -> (path=w3425:path)
            n2663 = call <vilib>:"Read Characters From File.vi"("file path (dialog if empty)"=w3425, "start of read offset (chars.:0)"=60 ("start of read offset (chars.: 0)")) -> ("character string"=→"String Control 2":string)  [unwired: 4 in, 3 out]
          }
        }
        n2664 = case shown="True" "OPEN 2" {
          frame False {
          }
          frame True {
            (unwired) 0  # existing file
            w3446 = "Choose a datalog file to open"  # prompt
            n2665 = local write "OPEN 2"(FALSE ("OPEN 1")) -> ()
            n2666 = String To Path(string="C:\\LAB-IQ\\Data\\") -> (path=w3431:path)
            n2667 = File Dialog(6:"*.dgf" ("pattern"), 7:w3446, 11:w3431) -> (0:w3429:errorcluster, 3:w3437:path)  [unwired: 4 in, 2 out]
            n2668 = Unbundle(w3429) -> ()  [unwired: 3 out]
            n2669 = Strip Path(path=w3437) -> (name=w3435:string)  [unwired: 1 out]
            n2670 = Path To String(path=w3437) -> (string=w3432:string)
            "string1 2" <- w3432
            n2671 = Match Pattern(string=w3435, regular expression=".dgf") -> (before substring=→"String Control 3":string)  [unwired: 1 in, 3 out]
            n2672 = Match Pattern(string=w3432, regular expression=".dgf" ("substring (\"\")")) -> (before substring=w3443:string)  [unwired: 1 in, 3 out]
            n2673 = Concatenate Strings(w3443, ".duf" ("Substring")) -> (w3440:string)
            n2674 = String To Path(string=w3440) -> (path=w3438:path)
            n2675 = call <vilib>:"Read Characters From File.vi"("file path (dialog if empty)"=w3438, "start of read offset (chars.:0)"=60 ("start of read offset (chars.: 0)")) -> ("character string"=→"String Control 4":string)  [unwired: 4 in, 3 out]
          }
        }
        n2676 = case shown="True" "OPEN 3" {
          frame False {
          }
          frame True {
            (unwired) 0  # existing file
            w3464 = "Choose a datalog file to open"  # prompt
            n2677 = local write "OPEN 3"(FALSE ("OPEN 1")) -> ()
            n2678 = String To Path(string="C:\\LAB-IQ\\Data\\") -> (path=w3449:path)
            n2679 = File Dialog(6:"*.dgf" ("pattern"), 7:w3464, 11:w3449) -> (0:w3447:errorcluster, 3:w3455:path)  [unwired: 4 in, 2 out]
            n2680 = Unbundle(w3447) -> ()  [unwired: 3 out]
            n2681 = Strip Path(path=w3455) -> (name=w3453:string)  [unwired: 1 out]
            n2682 = Path To String(path=w3455) -> (string=w3450:string)
            "string1 3" <- w3450
            n2683 = Match Pattern(string=w3453, regular expression=".dgf") -> (before substring=→"String Control 5":string)  [unwired: 1 in, 3 out]
            n2684 = Match Pattern(string=w3450, regular expression=".dgf" ("substring (\"\")")) -> (before substring=w3460:string)  [unwired: 1 in, 3 out]
            n2685 = Concatenate Strings(w3460, ".duf" ("Substring")) -> (w3457:string)
            n2686 = String To Path(string=w3457) -> (path=w3461:path)
            n2687 = call <vilib>:"Read Characters From File.vi"("file path (dialog if empty)"=w3461, "start of read offset (chars.:0)"=60 ("start of read offset (chars.: 0)")) -> ("character string"=→"String Control 6":string)  [unwired: 4 in, 3 out]
          }
        }
        n2688 = case shown="True" "OPEN 4" {
          frame False {
          }
          frame True {
            (unwired) 0  # existing file
            w3482 = "Choose a datalog file to open"  # prompt
            n2689 = local write "OPEN 4"(FALSE ("OPEN 1")) -> ()
            n2690 = String To Path(string="C:\\LAB-IQ\\Data\\") -> (path=w3467:path)
            n2691 = File Dialog(6:"*.dgf" ("pattern"), 7:w3482, 11:w3467) -> (0:w3465:errorcluster, 3:w3473:path)  [unwired: 4 in, 2 out]
            n2692 = Unbundle(w3465) -> ()  [unwired: 3 out]
            n2693 = Strip Path(path=w3473) -> (name=w3471:string)  [unwired: 1 out]
            n2694 = Path To String(path=w3473) -> (string=w3468:string)
            "string1 4" <- w3468
            n2695 = Match Pattern(string=w3471, regular expression=".dgf") -> (before substring=→"String Control 7":string)  [unwired: 1 in, 3 out]
            n2696 = Match Pattern(string=w3468, regular expression=".dgf" ("substring (\"\")")) -> (before substring=w3478:string)  [unwired: 1 in, 3 out]
            n2697 = Concatenate Strings(w3478, ".duf" ("Substring")) -> (w3475:string)
            n2698 = String To Path(string=w3475) -> (path=w3479:path)
            n2699 = call <vilib>:"Read Characters From File.vi"("file path (dialog if empty)"=w3479, "start of read offset (chars.:0)"=60 ("start of read offset (chars.: 0)")) -> ("character string"=→"String Control 8":string)  [unwired: 4 in, 3 out]
          }
        }
      }
      frame "About" {
        # "Elapsed time\ncof\nstroke\nmean pos\nTemp\nHumidity"
        n2700 = disable-structure shown="Disabled" {
          frame Disabled {
            n2701 = case shown="True" "Export" {
              frame False {
              }
              frame True {
                w3504 = "                                      " ("string")
                w3506 = "\r"
                (unwired) i16 6 ("width (-)")
                w3583 = "\r"
                w3515 = "\r"
                n2702 = local write "Export"(FALSE ("Export")) -> ()
                n2703 = local read "String 29"() -> (w3552:string)
                n2704 = local read "String 34"() -> (w3540:string)
                n2705 = local read "String 35"() -> (w3535:string)
                n2706 = local read "String 37"() -> (w3531:string)
                n2707 = local read "String 36"() -> (w3528:string)
                n2708 = local read "String 38"() -> (w3525:string)
                n2709 = local read "String 39"() -> (w3522:string)
